vi "RT Calibration.vi"(8 "error in (no error)":errorcluster, 10 "info":cluster{"File path":T2, "Cfg ":T3} {"Cfg"."Offset_rueda WS 2" format="%.27g"; "Cfg"."Offset_rueda WS 1" format="%.27g"; "Cfg"."Frecuencia de muestreo y módulo CRIO" items=["51.200 kS/s (NI 9234)"=1, "25.600 kS/s (NI 9234)"=2, "17.067 kS/s (NI 9234)"=3, "12.800 kS/s (NI 9234)"=4, "10.240 kS/s (NI 9234)"=5, "8.533 kS/s (NI 9234)"=6, "7.314 kS/s (NI 9234)"=7, "6.400 kS/s (NI 9234)"=8, "5.689 kS/s (NI 9234)"=9, "5.120 kS/s (NI 9234)"=10, "4.654 kS/s (NI 9234)"=11, "4.267 kS/s (NI 9234)"=12, "3.938 kS/s (NI 9234)"=13, "3.657 kS/s (NI 9234)"=14, "3.413 kS/s (NI 9234)"=15, "3.200 kS/s (NI 9234)"=16, "3.012 kS/s (NI 9234)"=17, "2.845 kS/s (NI 9234)"=18, "2.695 kS/s (NI 9234)"=19, "2.560 kS/s (NI 9234)"=20, "2.438 kS/s (NI 9234)"=21, "2.328 kS/s (NI 9234)"=22, "2.226 kS/s (NI 9234)"=23, "2.133 kS/s (NI 9234)"=24, "2.048 kS/s (NI 9234)"=25, "1.969 kS/s (NI 9234)"=26, "1.896 kS/s (NI 9234)"=27, "1.829 kS/s (NI 9234)"=28, "1.765 kS/s (NI 9234)"=29, "1.707 kS/s (NI 9234)"=30, "1.652 kS/s (NI 9234)"=31]}, 11 "Message Queues in":T5) -> (0 "error out":errorcluster)   [LabVIEW 2015]
uses:
  support/Message Queue/All Message Queues.ctl
  support/Message Queue/Message Cluster.ctl
  controls/File paths.ctl
  controls/Cfg_parameters.ctl
  <vilib>/LabVIEW Targets/FPGA/cRIO/shared/nicrio_ModuleControls/nicrio_cRIO-9234_DataRatesRing2.ctl
  controls/Calibration Data.ctl
  support/Message Queue/Enqueue Message (Single).vi
  <vilib>/Utility/config.llb/Write Key (Double).vi
  <vilib>/Utility/error.llb/Error Cluster From Error Code.vi
  <vilib>/ErrorRing/Error Ring.xnode
  support/Message Queue/Message Queue.lvlib
  <vilib>/Utility/config.llb/NI_LVConfig.lvlib
panel:
  out "mean":dbl format="%0.2f"
  in  "Calibration":T1
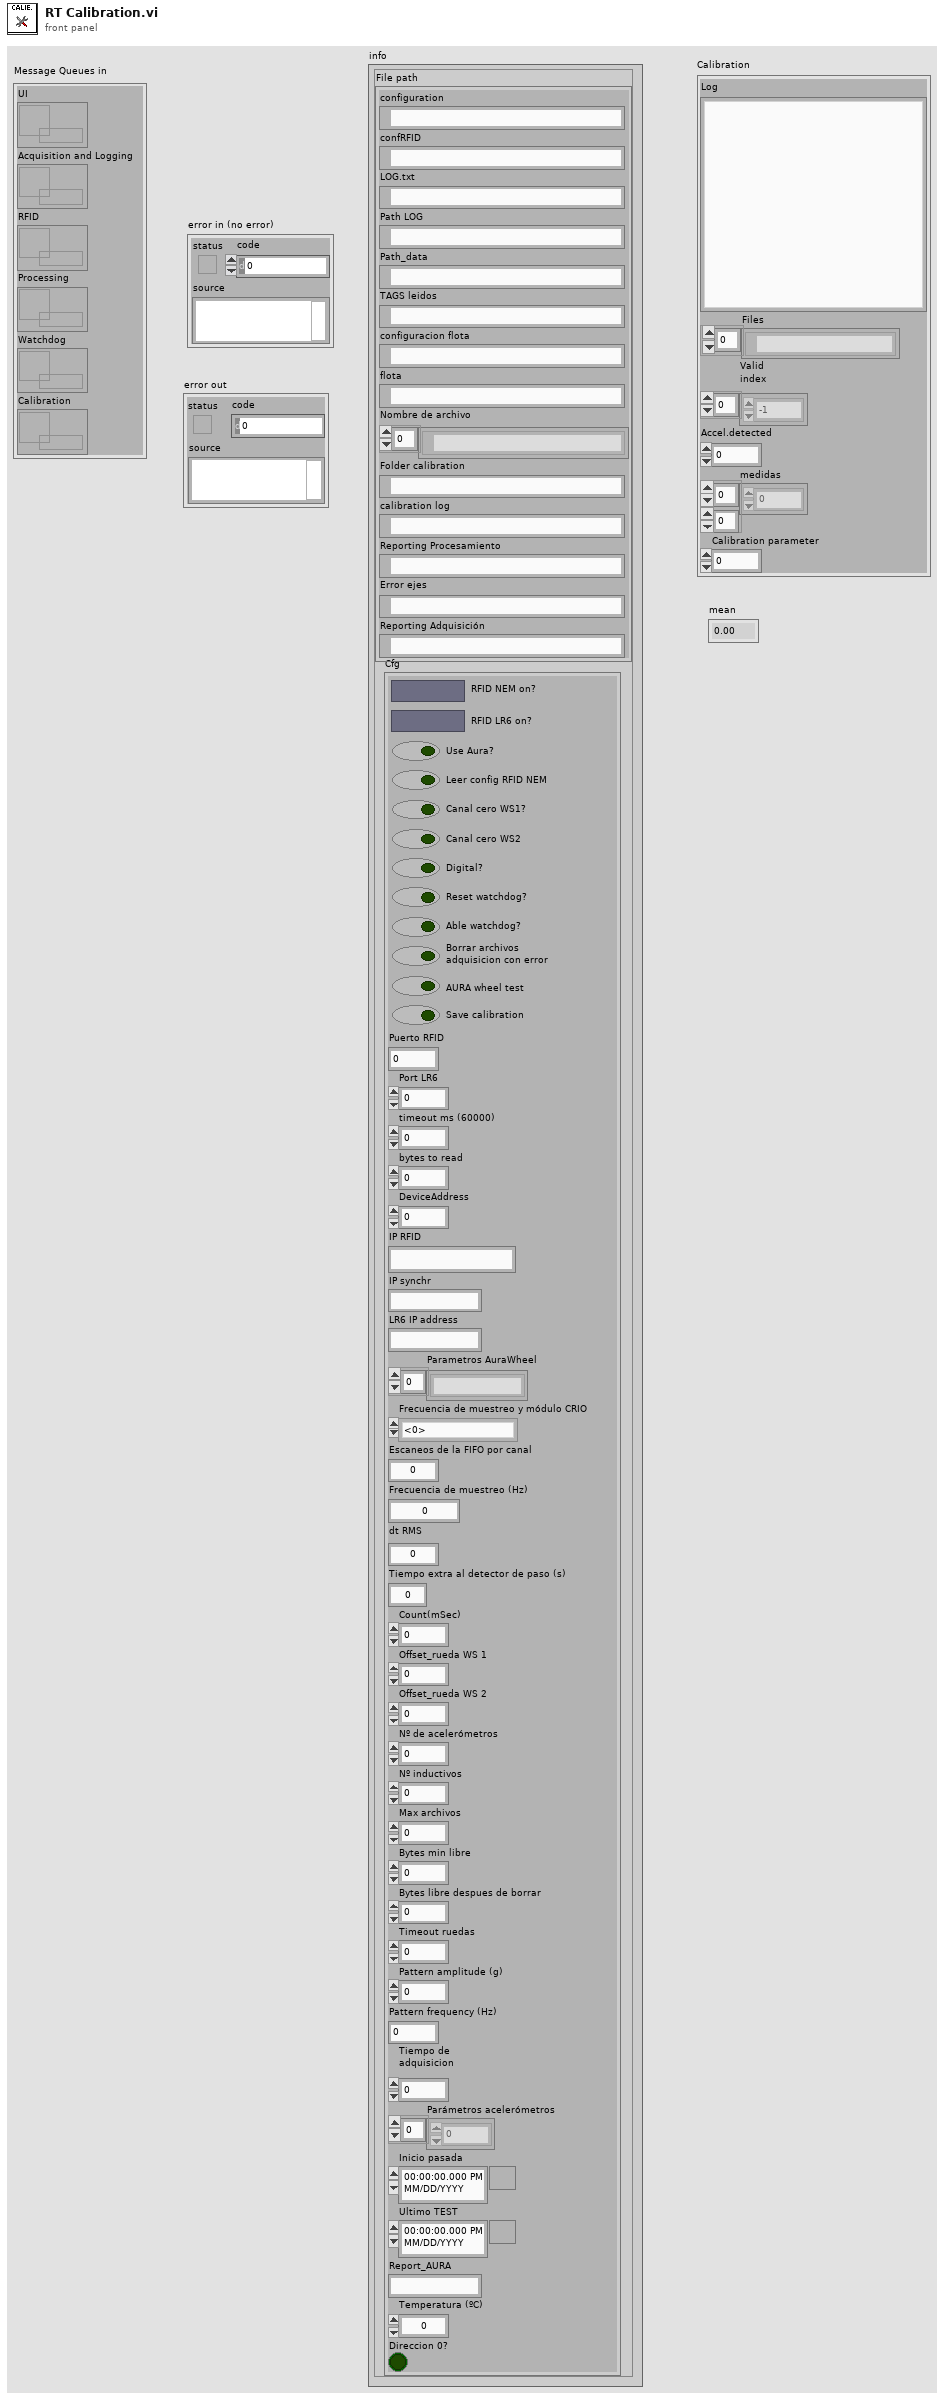
[diagram p1: front panel]
types:
  T1 = typedef "Calibration Data.ctl" = cluster{"Log":string, "Files":path[], "Valid\nindex":i32[], "Accel.detected":i32, "medidas":sgl[][], "Calibration parameter":dbl}
  T2 = typedef "File paths.ctl" = cluster{"configuration":path, "confRFID":path, "LOG.txt":path, "Path LOG":path, "Path_data":path, "TAGS leidos":path, "configuracion flota":path, "flota":path, "Nombre de archivo":path[], "Folder calibration":path, "calibration log":path, "Reporting Procesamiento":path, "Error ejes":path, "Reporting Adquisición":path}
  T3 = typedef "Cfg_parameters.ctl" = cluster{"RFID NEM on?":bool, "RFID LR6 on?":bool, "Use Aura?":bool, "Leer config RFID NEM":bool, "Canal cero WS1?":bool, "Canal cero WS2 ":bool, "Digital?":bool, "Reset watchdog?":bool, "Able watchdog?":bool, "Borrar archivos\nadquisicion con error":bool, "AURA wheel test":bool, "Save calibration":bool, "Puerto RFID":u16, "Port LR6":u16, "timeout ms (60000)":i32, "bytes to read":i32, "DeviceAddress":u8, "IP RFID":string, "IP synchr":string, "LR6 IP address":string, "Parametros AuraWheel":string[], "Frecuencia de muestreo y módulo CRIO":T4, "Escaneos de la FIFO por canal":u32, "Frecuencia de muestreo (Hz)":dbl, "dt RMS":dbl, "Tiempo extra al detector de paso (s)":dbl, "Count(mSec)":u32, "Offset_rueda WS 1":fxp<+/-,24,-4>, "Offset_rueda WS 2":fxp<+/-,24,-4>, "Nº de acelerómetros":i32, "Nº inductivos":i32, "Max archivos":u32, "Bytes min libre":u32, "Bytes libre despues de borrar":u32, "Timeout ruedas":dbl, "Pattern amplitude (g)":dbl, "Pattern frequency (Hz)":dbl, "Tiempo de adquisicion\n":dbl, "Parámetros acelerómetros":dbl[], "Inicio pasada":timestamp, "Ultimo TEST":timestamp, "Report_AURA":string, "Temperatura (ºC)":dbl, "Direccion 0?":bool}
  T4 = typedef "nicrio_cRIO-9234_DataRatesRing2.ctl" = u8
  T5 = typedef "Message Queue.lvlib/All Message Queues.ctl" = cluster{"UI":refnum<queue>, "Acquisition and Logging":refnum<queue>, "RFID":refnum<queue>, "Processing":refnum<queue>, "Watchdog":refnum<queue>, "Calibration":refnum<queue>}
  T6 = typedef "NI_LVConfig.lvlib/Config Data RefNum.ctl" = refnum<k1>
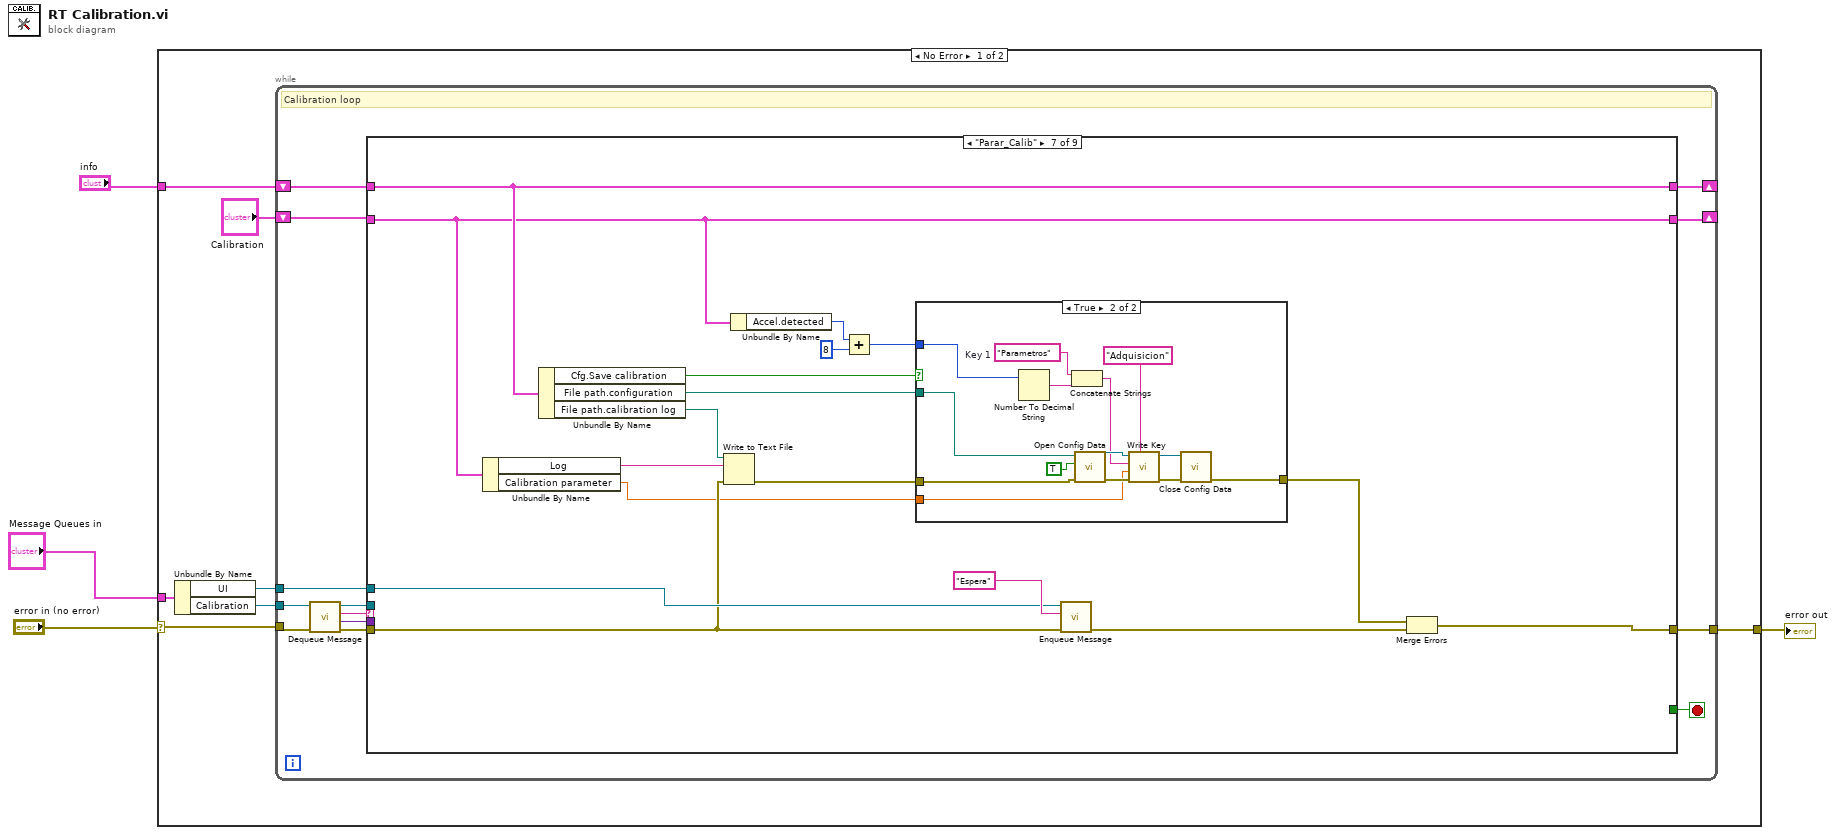
[diagram p0: block diagram]
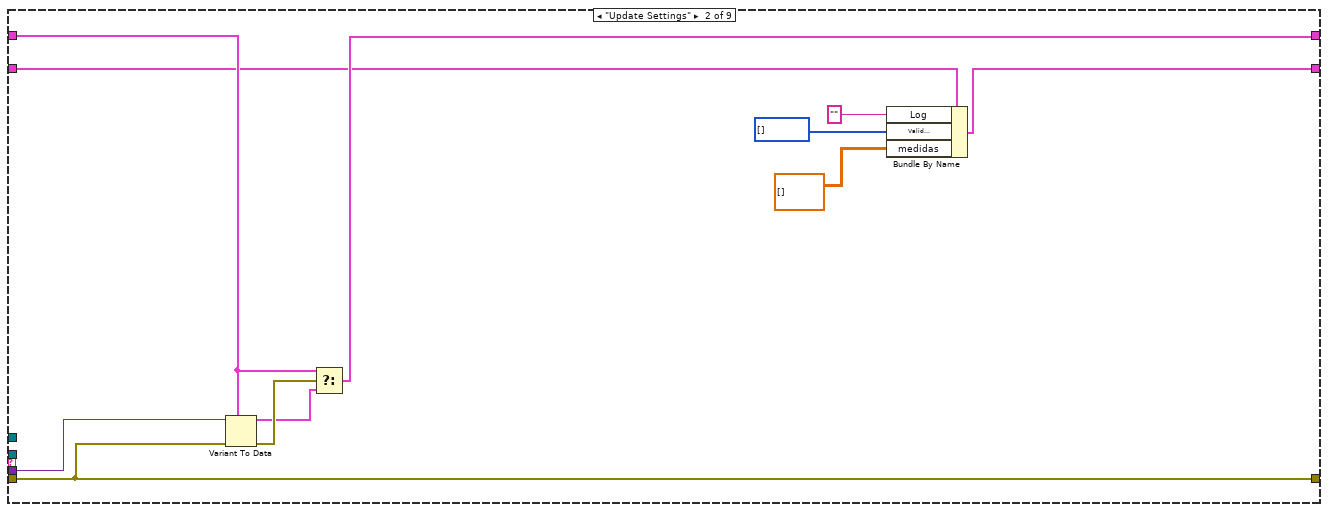
[diagram p3: hidden frame]
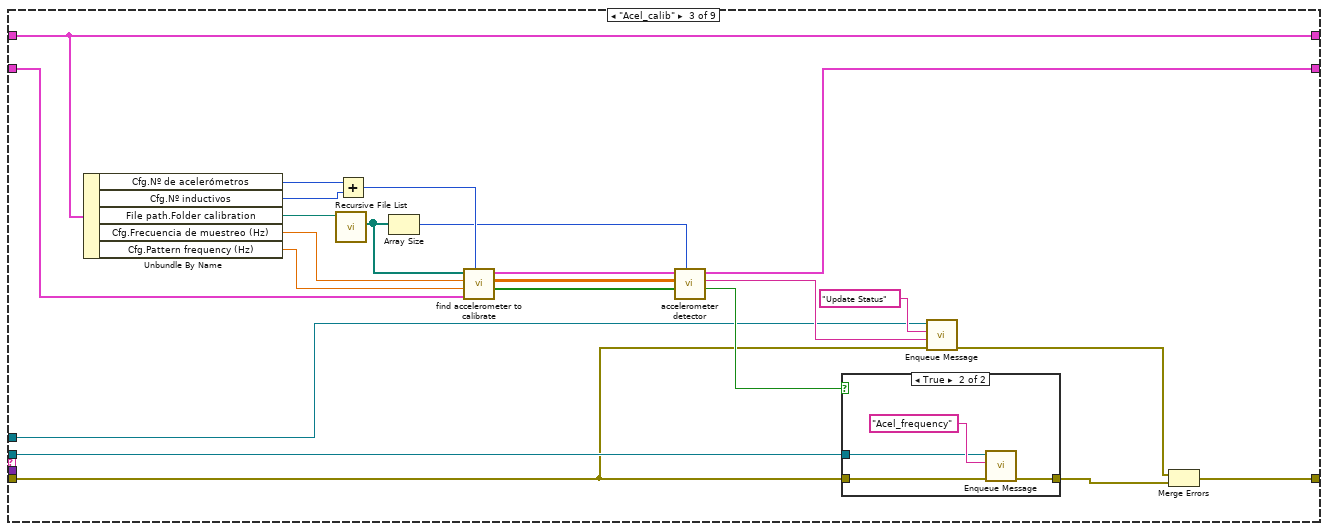
[diagram p4: hidden frame]
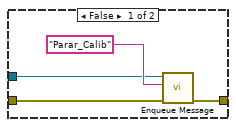
[diagram p5: hidden frame]
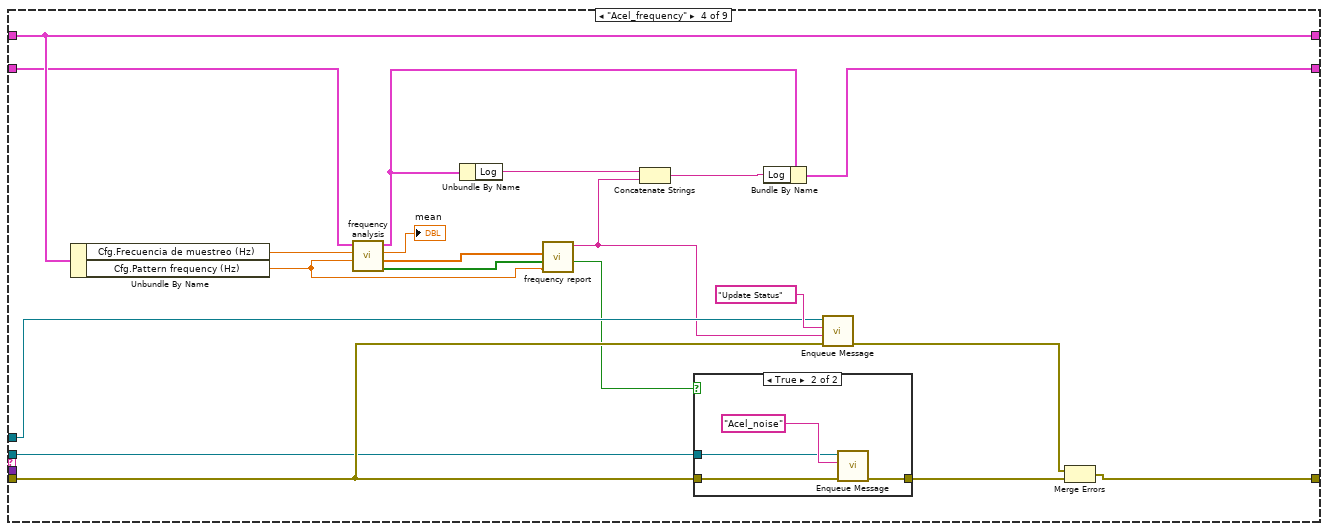
[diagram p6: hidden frame]
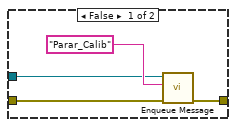
[diagram p7: hidden frame]
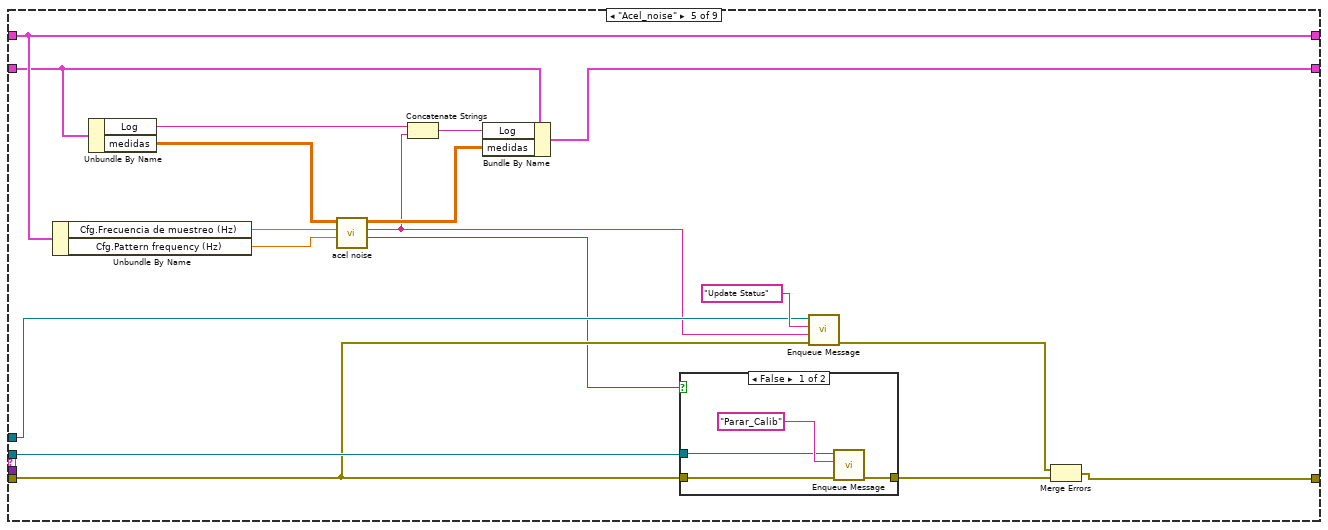
[diagram p8: hidden frame]
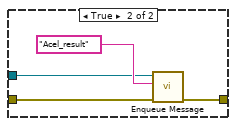
[diagram p9: hidden frame]
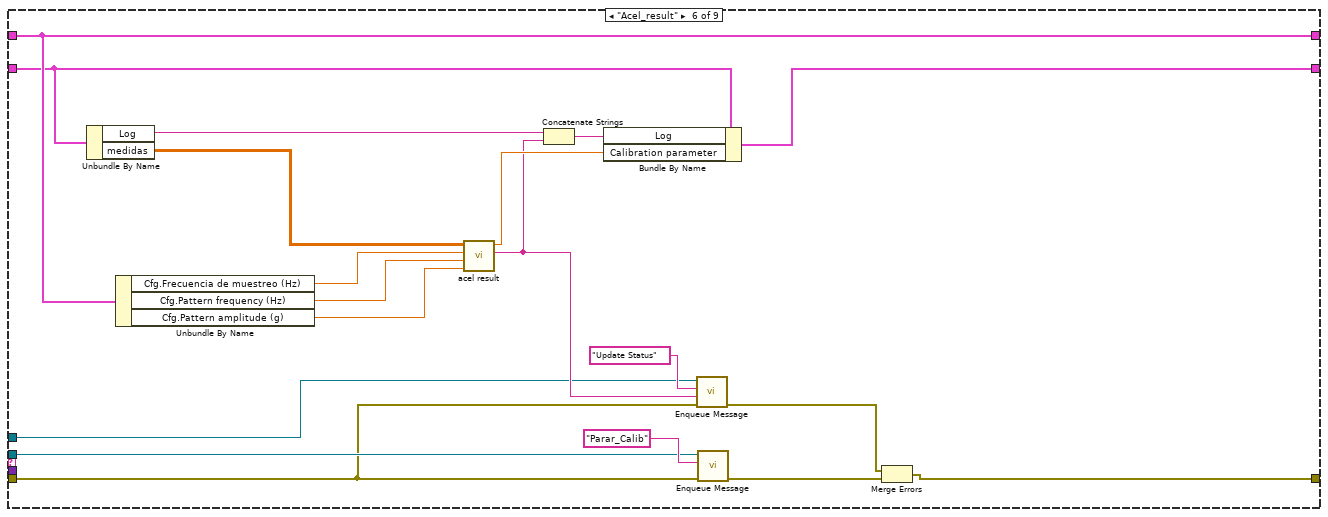
[diagram p10: hidden frame]
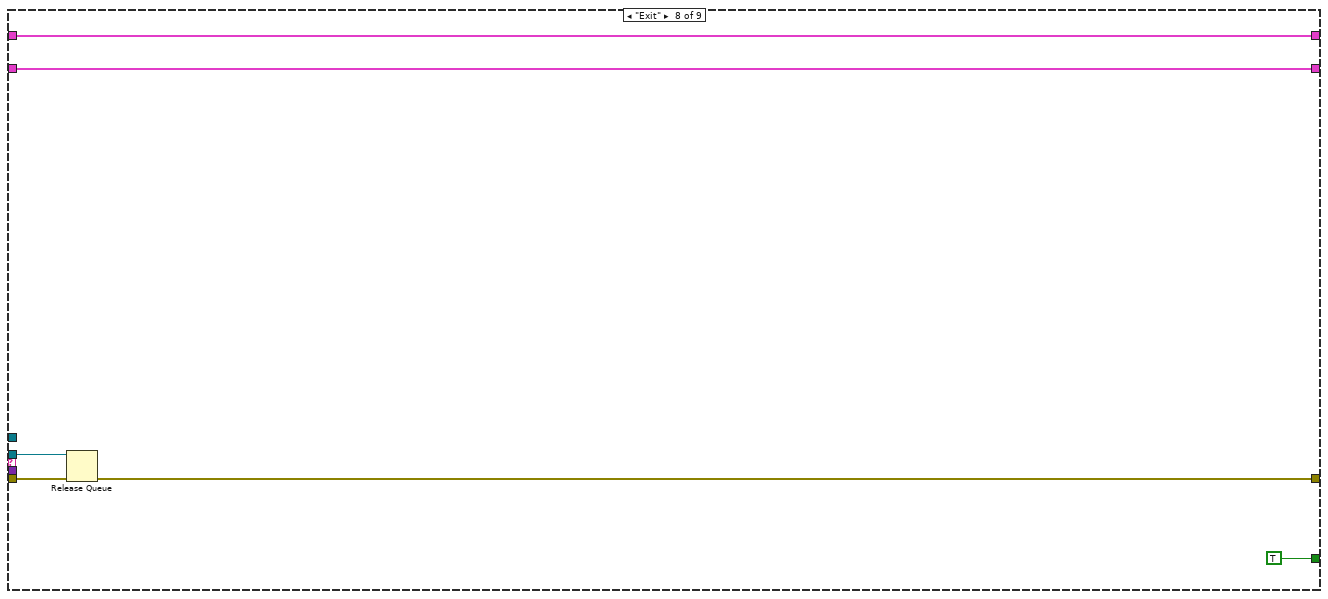
[diagram p12: hidden frame]
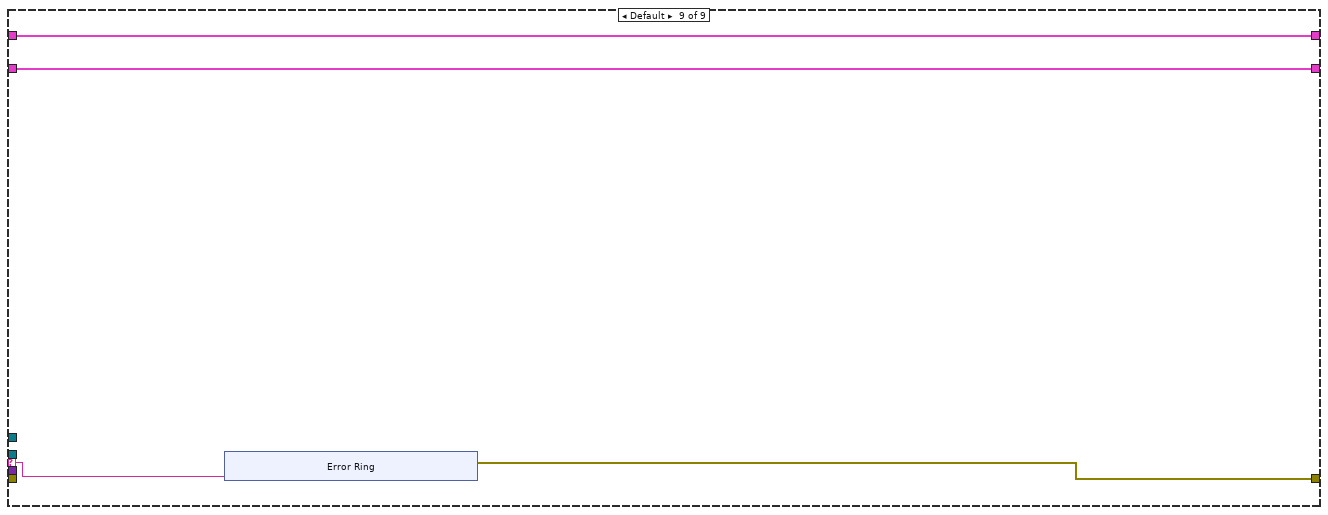
[diagram p13: hidden frame]
diagram:
  n1 = case shown="No Error" "error in (no error)" {
    selector: "error in (no error)" -> [w10 w192]
    tunnel: "Message Queues in" -> [w11 _]
    tunnel: "info" -> [w7 _]
    tunnel: [w6 w192] -> w1
    frame No Error {
      n2 = Unbundle By Name(w11) -> ("UI"=w8:refnum<queue>, "Calibration"=w9:refnum<queue>)
      n3 = while {
        tunnel: w10 -> [w24]
        tunnel: w9 -> [w23]
        tunnel: w8 -> [w21]
        shift-right: [w17] -> _
        shift-left: w7 -> [w18]
        tunnel: [w15] -> w6
        shift-right: [w12] -> _
        shift-left: "Calibration" -> [w13]
        stop <- w16 stop-if-true
        # "Calibration loop"
        n4 = call "Dequeue Message.vi"("error in (no error)"=w24, "Message Queue"=w23) -> ("error out"=w20:errorcluster, "Message Data"=w14:variant, "Message"=w19:string, "dup Message Queue"=w22:refnum<queue>)  [unwired: 6 in]
        n5 = case shown="\"Parar_Calib\"" w19 {
          selector: w19 -> [_ _ _ _ _ _ _ _ w182]
          tunnel: w22 -> [_ _ w43 w71 w103 w140 _ w178 _]
          tunnel: w21 -> [_ _ w44 w73 w102 w128 w158 _ _]
          tunnel: w20 -> [w27 w35 w42 w74 w101 w127 w148 w179 _]
          tunnel: [w27 w35 w41 w75 w104 w124 w145 w177 w183] -> w15
          tunnel: w18 -> [w26 w34 w61 w88 w115 w142 w156 w180 w184]
          tunnel: [w26 w33 w61 w88 w115 w142 w156 w180 w184] -> w17
          tunnel: [_ _ _ _ _ _ _ TRUE _] -> w16
          tunnel: w14 -> [_ w38 _ _ _ _ _ _ _]
          tunnel: w13 -> [w25 w32 w53 w82 w111 w135 w154 w175 w181]
          tunnel: [w25 w31 w48 w79 w98 w130 w154 w175 w181] -> w12
          frame "Initialize" {
          }
          frame "Update Settings" {
            n6 = Variant To Data(error in=w35, type=w34, Variant=w38) -> (data=w36:cluster{"File path":T2, "Cfg ":T3}, error out=w37:errorcluster)
            n7 = Select(t=w34, s=w37, f=w36) -> (s? t:f=w33:cluster{"File path":T2, "Cfg ":T3})
            n8 = Bundle By Name(cluster=w32, "Log"="", "Valid\nindex"=i32[] [], "medidas"=sgl[][] []) -> (w31:T1)
          }
          frame "Acel_calib" {
            n9 = Unbundle By Name(w61) -> ("Cfg.Nº de acelerómetros"=w56:i32, "Cfg.Nº inductivos"=w55:i32, "File path.Folder calibration"=w60:path, "Cfg.Frecuencia de muestreo (Hz)"=w58:dbl, "Cfg.Pattern frequency (Hz)"=w57:dbl)
            n10 = call <vilib>:"Recursive File List.vi"("Folder Path"=w60) -> ("All Files in Dir"=w59:path[])  [unwired: 6 in, 4 out]
            n11 = Add(x=w56, y=w55) -> (x+y=w54:i32)
            n12 = Array Size(array=w59) -> (size(s)=w49:i32)
            n13 = call "find accelerometer to calibrate.vi"("All Files in Dir"=w59, "Frecuencia de muestreo (Hz)"=w58, "Pattern frequency (Hz)"=w57, "Calibration"=w53, "Elementos"=w54) -> ("Calibration out"=w52:T1, "Data"=w51:sgl[][][], "1 accel found?"=w50:bool[])  [unwired: 3 in]
            n14 = call "accelerometer detector.vi"("Calibration"=w52, "Data"=w51, "1 accel found?"=w50, "Nº meas"=w49) -> ("output cluster"=w48:T1, "report"=w45:string, "Continuar?"=w47:bool)  [unwired: 4 in]
            n15 = case shown="True" w47 {
              tunnel: w42 -> [w64 w68]
              tunnel: [w63 w67] -> w39
              tunnel: w43 -> [w62 w66]
              frame False {
                n16 = call-poly "Enqueue Message.vi"("error in (no error)"=w64, "Message"="Parar_Calib", "Message Queue"=w62) -> ("error out"=w63:errorcluster)  [unwired: 7 in, 1 out]
              }
              frame True {
                n17 = call-poly "Enqueue Message.vi"("error in (no error)"=w68, "Message"="Acel_frequency", "Message Queue"=w66) -> ("error out"=w67:errorcluster)  [unwired: 7 in, 1 out]
              }
            }
            n18 = call-poly "Enqueue Message.vi"("error in (no error)"=w42, "Message Data"=w45, "Message"="Update Status", "Message Queue"=w44) -> ("error out"=w40:errorcluster)  [unwired: 6 in, 1 out]
            n19 = Merge Errors(w40, w39) -> (w41:errorcluster)
          }
          frame "Acel_frequency" {
            n20 = Unbundle By Name(w88) -> ("Cfg.Frecuencia de muestreo (Hz)"=w87:dbl, "Cfg.Pattern frequency (Hz)"=w86:dbl)
            n21 = call "frequency analysis.vi"("Pattern frequency (Hz)"=w86, "Frecuencia de muestreo (Hz)"=w87, "Calibration"=w82) -> ("Frecuencias validas"=w84:bool[], "Magnitude*df"=w85:dbl[], "mean"=→"mean":dbl, "output calibration"=w80:T1)  [unwired: 5 in]
            n22 = Unbundle By Name(w80) -> ("Log"=w83:string)
            n23 = call "frequency report.vi"("Pattern frequency (Hz)"=w86, "Frecuencias validas"=w84, "Magnitud*df"=w85) -> ("continuar?"=w70:bool, "Report"=w72:string)  [unwired: 7 in]
            n24 = Concatenate Strings(w83, w72) -> (w81:string)
            n25 = case shown="True" w70 {
              tunnel: w74 -> [w92 w96]
              tunnel: [w91 w95] -> w76
              tunnel: w71 -> [w90 w94]
              frame False {
                n26 = call-poly "Enqueue Message.vi"("error in (no error)"=w92, "Message"="Parar_Calib", "Message Queue"=w90) -> ("error out"=w91:errorcluster)  [unwired: 7 in, 1 out]
              }
              frame True {
                n27 = call-poly "Enqueue Message.vi"("error in (no error)"=w96, "Message"="Acel_noise", "Message Queue"=w94) -> ("error out"=w95:errorcluster)  [unwired: 7 in, 1 out]
              }
            }
            n28 = Bundle By Name(cluster=w80, "Log"=w81) -> (w79:T1)
            n29 = call-poly "Enqueue Message.vi"("error in (no error)"=w74, "Message Data"=w72, "Message"="Update Status", "Message Queue"=w73) -> ("error out"=w77:errorcluster)  [unwired: 6 in, 1 out]
            n30 = Merge Errors(w77, w76) -> (w75:errorcluster)
          }
          frame "Acel_noise" {
            n31 = Unbundle By Name(w115) -> ("Cfg.Frecuencia de muestreo (Hz)"=w113:dbl, "Cfg.Pattern frequency (Hz)"=w112:dbl)
            n32 = Unbundle By Name(w111) -> ("Log"=w110:string, "medidas"=w114:sgl[][])
            n33 = call "acel noise.vi"("Pattern frequency (Hz)"=w112, "Frecuencia de muestreo (Hz)"=w113, "medidas"=w114) -> ("Continuar?"=w99:bool, "Report"=w100:string, "medidas out"=w108:sgl[][])  [unwired: 6 in]
            n34 = Concatenate Strings(w110, w100) -> (w109:string)
            n35 = Bundle By Name(cluster=w111, "Log"=w109, "medidas"=w108) -> (w98:T1)
            n36 = case shown="False" w99 {
              tunnel: w101 -> [w118 w122]
              tunnel: [w117 w121] -> w105
              tunnel: w103 -> [w116 w120]
              frame False {
                n37 = call-poly "Enqueue Message.vi"("error in (no error)"=w118, "Message"="Parar_Calib", "Message Queue"=w116) -> ("error out"=w117:errorcluster)  [unwired: 7 in, 1 out]
              }
              frame True {
                n38 = call-poly "Enqueue Message.vi"("error in (no error)"=w122, "Message"="Acel_result", "Message Queue"=w120) -> ("error out"=w121:errorcluster)  [unwired: 7 in, 1 out]
              }
            }
            n39 = call-poly "Enqueue Message.vi"("error in (no error)"=w101, "Message Data"=w100, "Message"="Update Status", "Message Queue"=w102) -> ("error out"=w106:errorcluster)  [unwired: 6 in, 1 out]
            n40 = Merge Errors(w106, w105) -> (w104:errorcluster)
          }
          frame "Acel_result" {
            n41 = Unbundle By Name(w135) -> ("Log"=w133:string, "medidas"=w139:sgl[][])
            n42 = Unbundle By Name(w142) -> ("Cfg.Frecuencia de muestreo (Hz)"=w138:dbl, "Cfg.Pattern frequency (Hz)"=w137:dbl, "Cfg.Pattern amplitude (g)"=w136:dbl)
            n43 = call "acel result.vi"("Pattern amplitude"=w136, "Pattern frequency (Hz)"=w137, "Frecuencia de muestreo (Hz)"=w138, "medidas"=w139) -> ("Report"=w129:string, "Calibration parameter"=w132:dbl)  [unwired: 6 in]
            n44 = Concatenate Strings(w133, w129) -> (w134:string)
            n45 = Bundle By Name(cluster=w135, "Log"=w134, "Calibration parameter"=w132) -> (w130:T1)
            n46 = call-poly "Enqueue Message.vi"("error in (no error)"=w127, "Message Data"=w129, "Message"="Update Status", "Message Queue"=w128) -> ("error out"=w126:errorcluster)  [unwired: 6 in, 1 out]
            n47 = call-poly "Enqueue Message.vi"("error in (no error)"=w127, "Message"="Parar_Calib", "Message Queue"=w140) -> ("error out"=w125:errorcluster)  [unwired: 7 in, 1 out]
            n48 = Merge Errors(w126, w125) -> (w124:errorcluster)
          }
          frame "Parar_Calib" {
            n49 = Unbundle By Name(w154) -> ("Log"=w157:string, "Calibration parameter"=w146:dbl)
            n50 = Unbundle By Name(w156) -> ("Cfg.Save calibration"=w151:bool, "File path.configuration"=w149:path, "File path.calibration log"=w155:path)
            n51 = Write to Text File(file (use dialog)=w155, text=w157, error in=w148) -> (error out=w147:errorcluster)  [unwired: 1 in, 2 out]
            n52 = Unbundle By Name(w154) -> ("Accel.detected"=w152:i32)
            n53 = Add(x=w152, y=8) -> (x+y=w150:i32)
            n54 = case shown="True" w151 {
              tunnel: w150 -> [_ w165]
              tunnel: w149 -> [_ w164]
              tunnel: w147 -> [w160 w163]
              tunnel: [w160 w162] -> w144
              tunnel: w146 -> [_ w161]
              frame False {
              }
              frame True {
                w173 = "Parametros"  # Key 1
                n55 = Number To Decimal String(number=w165) -> (decimal integer string=w174:string)  [unwired: 1 in]
                n56 = Concatenate Strings(w173, w174) -> (w167:string)
                n57 = call <vilib>:"Open Config Data.vi"("error in (no error)"=w163, "create file if necessary (T)"=TRUE, "configuration file path"=w164) -> ("error out"=w168:errorcluster, "refnum"=w169:T6)  [unwired: 7 out]
                n58 = call-poly <vilib>:"Write Key.vi"("section"="Adquisicion", "error in (no error)"=w168, "value"=w161, "key"=w167, "refnum"=w169) -> ("error out"=w172:errorcluster, "refnum out"=w171:T6)  [unwired: 3 in, 2 out]
                n59 = call <vilib>:"Close Config Data.vi"("error in (no error)"=w172, "refnum"=w171) -> ("error out"=w162:errorcluster)  [unwired: 8 in, 1 out]
              }
            }
            n60 = call-poly "Enqueue Message.vi"("error in (no error)"=w148, "Message"="Espera", "Message Queue"=w158) -> ("error out"=w143:errorcluster)  [unwired: 7 in, 1 out]
            n61 = Merge Errors(w144, w143) -> (w145:errorcluster)
          }
          frame "Exit" {
            n62 = Release Queue(queue=w178, error in (no error)=w179) -> (error out=w177:errorcluster)  [unwired: 1 in, 2 out]
          }
          frame Default {
            n63 = xnode "Error Ring"("parameter 0"=w182) -> ("error out"=w183:errorcluster)
          }
        }
      }
    }
    frame Error {
    }
  }
  "error out" <- w1
